vi "temp--set tags.vi"() -> ()   [LabVIEW 2015]
doc: "Temporary helper VI to apply user tags to the controls in the project so that they can be used with the TSC Material Toolkit.\n\n<b>Code Developed By:</b>\nTechnology Service Corporation\nBloomington, IN 47403\nwww.tsc.com/atcs\n\nDeveloper:\nDaniel Coons"
panel:
  out "error out":errorcluster
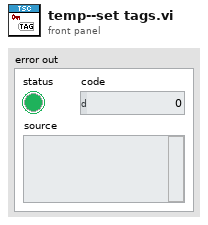
[diagram p1: front panel]
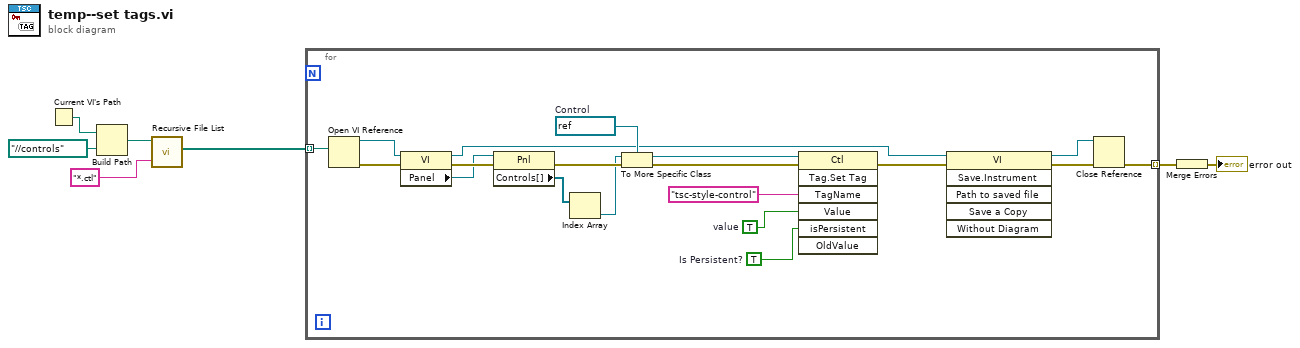
[diagram p0: block diagram]
diagram:
  n1 = Current VI's Path() -> (path=w7:path)
  n2 = Build Path(base path=w7, name or relative path=path "../../controls") -> (appended path=w5:path)
  n3 = call <vilib>:"Recursive File List.vi"("pattern"="*.ctl", "Folder Path"=w5) -> ("All Files in Dir"=w1:path[])  [unwired: 5 in, 4 out]
  n4 = for {
    tunnel: w1 -> [w23] mode=indexing
    tunnel: [w25] -> w3 mode=indexing
    w11 = TRUE  # Is Persistent?
    w12 = TRUE  # value
    w14 = refnum<vi> refnum  # Control
    n5 = Open VI Reference(vi path=w23) -> (vi reference=w21:refnum<vi>, error out=w26:errorcluster)  [unwired: 5 in]
    n6 = property class="VI"(reference=w21, error in=w26) -> (reference out=w9:refnum<vi>, error out=w20:errorcluster, "Panel"=w18:refnum<vi>)
    n7 = property class="Pnl"(reference=w18, error in=w20) -> (error out=w19:errorcluster, "Controls[]"=w17:refnum<vi>[])  [unwired: 1 out]
    n8 = Index Array(array=w17) -> (element=w15:refnum<vi>)  [unwired: 1 in]
    n9 = To More Specific Class(target class=w14, reference=w15, error in=w19) -> (specific class reference=w13:refnum<vi>, error out=w16:errorcluster)
    n10 = invoke class="Ctl" method="Tag.Set Tag"(reference=w13, error in=w16, "TagName"="tsc-style-control" ("Tag Name"), "Value"=w12, "isPersistent"=w11) -> (error out=w24:errorcluster)  [unwired: 2 in, 6 out]
    n11 = invoke class="VI" method="Save.Instrument"(reference=w9, error in=w24) -> (reference out=w8:refnum<vi>, error out=w10:errorcluster)  [unwired: 4 in, 4 out]
    n12 = Close Reference(reference=w8, error in (no error)=w10) -> (error out=w25:errorcluster)
  }
  n13 = Merge Errors(w3) -> (→"error out":errorcluster)
